vi "Add Controls to Method.vi"(8 "error in (no error)":errorcluster, 10 "Controls in":refnum<vi>[](array[refnum]), 11 "vi ref in":refnum<vi>) -> (0 "error out":errorcluster, 2 "Controls out":refnum<vi>[](array[refnum]), 3 "vi ref out":refnum<vi>)   [LabVIEW 2020, in "Message Maker.lvlib"]
uses:
  Message Maker.lvlib
  <vilib>/Utility/miscctls.llb/LVPositionTypeDef.ctl
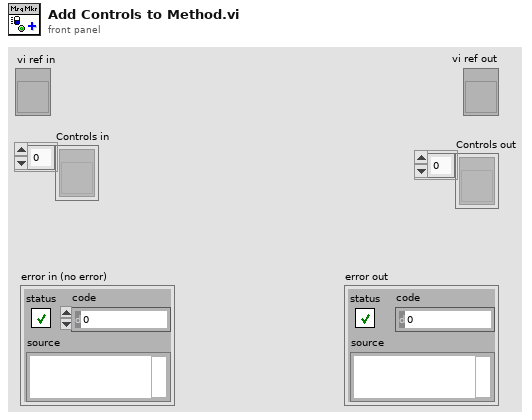
[diagram p1: front panel]
types:
  T1 = typedef "LVPositionTypeDef.ctl" = cluster{"Left":i32, "Top":i32}
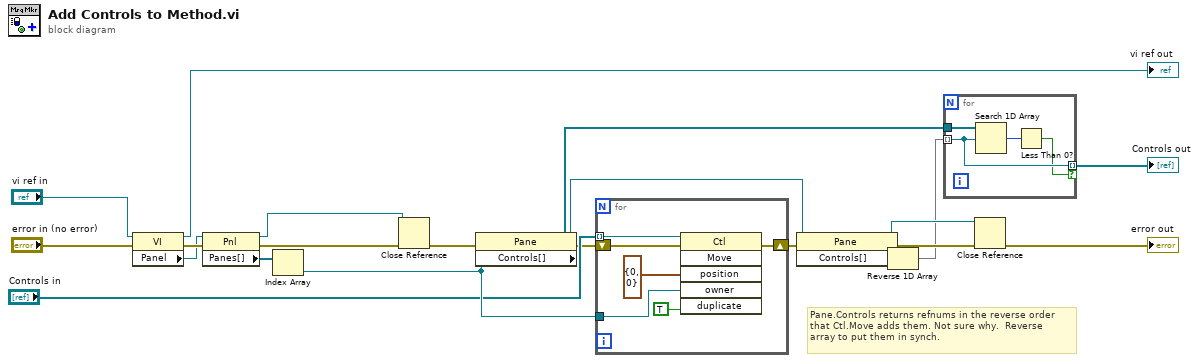
[diagram p0: block diagram]
diagram:
  # "Pane.Controls returns refnums in the reverse order\nthat Ctl.Move adds them. Not sure why.  Reverse\narray to put them in synch."
  n1 = property class="VI"(reference="vi ref in", error in="error in (no error)") -> (reference out=→"vi ref out":refnum<vi>, error out=w16:errorcluster, "Panel"=w15:refnum<vi>)
  n2 = property class="Pnl"(reference=w15, error in=w16) -> (reference out=w21:refnum<vi>, error out=w17:errorcluster, "Panes[]"=w13:refnum<vi>[])
  n3 = Index Array(array=w13) -> (element=w14:refnum<vi>)  [unwired: 1 in]
  n4 = Close Reference(reference=w21, error in (no error)=w17) -> (error out=w3:errorcluster)
  n5 = property class="Pane"(reference=w14, error in=w3) -> (reference out=w6:refnum<vi>, error out=w7:errorcluster, "Controls[]"=w4:refnum<vi>[])
  n6 = for {
    tunnel: "Controls in" -> [w27] mode=indexing
    shift-right: [w24] -> w9
    shift-left: w7 -> [w25]
    tunnel: w14 -> [w22]
    n7 = invoke class="Ctl" method="Move"(reference=w27, error in=w25, "position"=T1 {"Left"=0, "Top"=0}, "owner"=w22, "duplicate"=TRUE ("Duplicate? (F)")) -> (error out=w24:errorcluster)  [unwired: 1 in, 5 out]
  }
  n8 = property class="Pane"(reference=w6, error in=w9) -> (reference out=w2:refnum<vi>, error out=w8:errorcluster, "Controls[]"=w5:refnum<vi>[])
  n9 = Reverse 1D Array(array=w5) -> (reversed array=w1:refnum<vi>[])
  n10 = for {
    tunnel: w1 -> [w30] mode=indexing
    tunnel: w4 -> [w31]
    tunnel: [w30] -> w12 mode=indexing if=w28
    n11 = Search 1D Array(1D array=w31, element=w30) -> (index of element=w29:i32)  [unwired: 1 in]
    n12 = Less Than 0?(x=w29) -> (x < 0?=w28:bool)
  }
  "Controls out" <- w12
  n13 = Close Reference(reference=w2, error in (no error)=w8) -> (error out=→"error out":errorcluster)
